vi "LogData.vi"(8 "error in":errorcluster, 10 "Data_Cluster":T1 {"Coil Temperature" format="%.2f"; "Channel 2 (c2)" format="%.3f"; "Channel 1 (c1)" format="%.3f"; "Freqency +45 Deg" format="%.7f"; "Freqency -45 Deg" format="%.7f"; "Freqency 0 Deg" format="%.7f"; "df frequency quotient" format="%.7f"; "Density" format="%.3f"; "Viscosity" format="%.3f"; "Damping Frequency" format="%.2g"; "Resonant Frequency" format="%.2f"; "Temperature" format="%.2f"}) -> (0 "error out":errorcluster)   [LabVIEW 2019, in "SME_Data_Acquisition.lvlib"]
doc: "This even is generated by helper loop to log data.\n_____\nCreated using DQMH Event Scripter 7.0.1.1316."
uses:
  SME_Data_Acquisition.lvlib
  LogData Argument--cluster.ctl
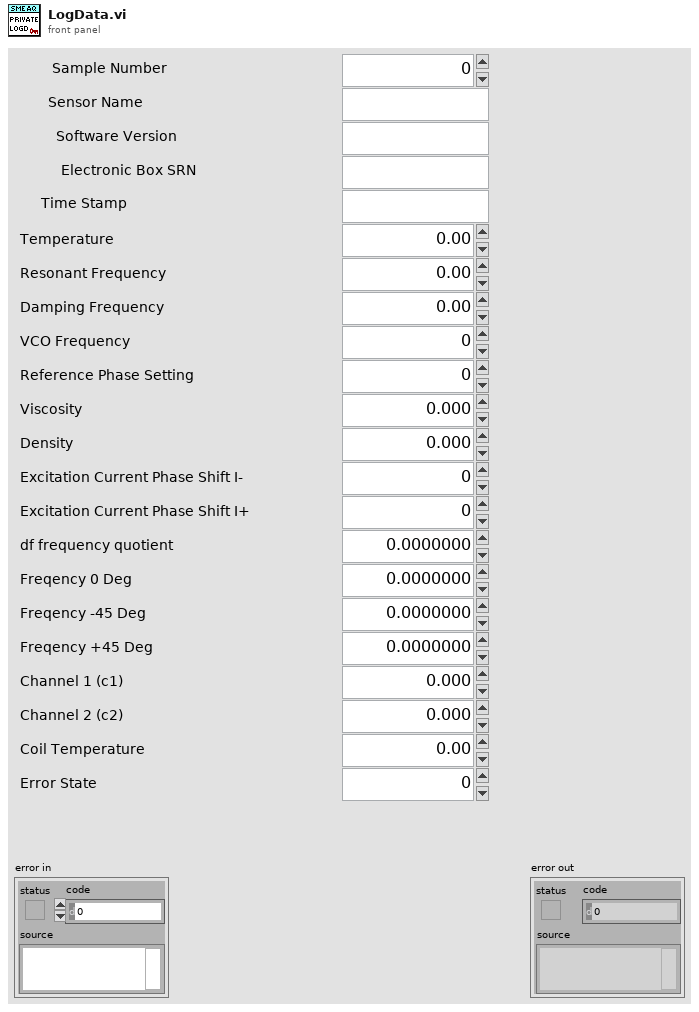
[diagram p1: front panel]
types:
  T1 = cluster{"Sample Number":u16, "Sensor Name":string, "Software Version":string, "Electronic Box SRN":string, "Time Stamp":string, "Temperature":dbl, "Resonant Frequency":dbl, "Damping Frequency":dbl, "VCO Frequency":u16, "Reference Phase Setting":u16, "Viscosity":dbl, "Density":dbl, "Excitation Current Phase Shift I-":u16, "Excitation Current Phase Shift I+":u16, "df frequency quotient":dbl, "Freqency 0 Deg":dbl, "Freqency -45 Deg":dbl, "Freqency +45 Deg":dbl, "Channel 1 (c1)":dbl, "Channel 2 (c2)":dbl, "Coil Temperature":dbl, "Error State":u8}
  T2 = typedef "SME_Data_Acquisition.lvlib/LogData Argument--cluster.ctl" = cluster{"Data_Cluster":cluster{"Sample Number":u16, "Sensor Name":string, "Software Version":string, "Electronic Box SRN":string, "Time Stamp":string, "Temperature":dbl, "Resonant Frequency":dbl, "Damping Frequency":dbl, "VCO Frequency":u16, "Reference Phase Setting":u16, "Viscosity":dbl, "Density":dbl, "Excitation Current Phase Shift I-":u16, "Excitation Current Phase Shift I+":u16, "df frequency quotient":dbl, "Freqency 0 Deg":dbl, "Freqency -45 Deg":dbl, "Freqency +45 Deg":dbl, "Channel 1 (c1)":dbl, "Channel 2 (c2)":dbl, "Coil Temperature":dbl, "Error State":u8}}
  T3 = typedef "SME_Data_Acquisition.lvlib/Request Events--cluster.ctl" = cluster{"Stop Module":refnum<user-event>, "Show Panel":refnum<user-event>, "Hide Panel":refnum<user-event>, "Get Module Execution Status":refnum<user-event>, "Show Diagram":refnum<user-event>, "Private":cluster{"LogData":refnum<user-event>}}
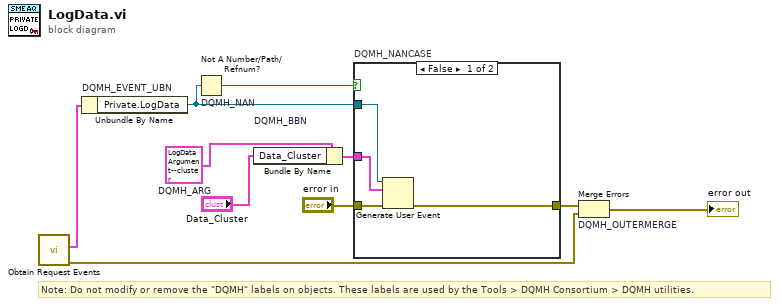
[diagram p0: block diagram]
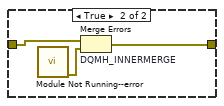
[diagram p2: hidden frame]
diagram:
  w4 = T2 {"Data_Cluster"={"Sample Number"=0, "Sensor Name"="", "Software Version"="", "Electronic Box SRN"="", "Time Stamp"="", "Temperature"=0.0, "Resonant Frequency"=0.0, "Damping Frequency"=0.0, "VCO Frequency"=0, "Reference Phase Setting"=0, "Viscosity"=0.0, "Density"=0.0, "Excitation Current Phase Shift I-"=0, "Excitation Current Phase Shift I+"=0, "df frequency quotient"=0.0, "Freqency 0 Deg"=0.0, "Freqency -45 Deg"=0.0, "Freqency +45 Deg"=0.0, "Channel 1 (c1)"=0.0, "Channel 2 (c2)"=0.0, "Coil Temperature"=0.0, "Error State"=0}}  # DQMH_ARG
  # "Note: Do not modify or remove the \"DQMH\" labels on objects. These labels are used by the Tools > DQMH Consortium > DQMH utilities."
  n1 = call "Obtain Request Events.vi"() -> ("error out"=w2:errorcluster, "SME_Data_Acquisition Request Events"=w1:T3)  [unwired: 10 in]
  n2 = Unbundle By Name "DQMH_EVENT_UBN"(w1) -> ("Private.LogData"=w6:refnum<user-event>)
  n3 = Not A Number/Path/Refnum? "DQMH_NAN"(number/path/refnum=w6) -> (NaN/Path/Refnum?=w7:bool)
  n4 = Bundle By Name "DQMH_BBN"(cluster=w4, "Data_Cluster"="Data_Cluster") -> (w8:T2)
  n5 = case "DQMH_NANCASE" shown="False" w7 {
    tunnel: "error in" -> [w14 w17]
    tunnel: [w13 w16] -> w5
    tunnel: w6 -> [w12 _]
    tunnel: w8 -> [w11 _]
    frame False {
      n6 = Generate User Event(user event=w12, event data cluster=w11, error in=w14) -> (error out=w13:errorcluster)  [unwired: 1 in, 1 out]
    }
    frame True {
      n7 = call "Module Not Running--error.vi"() -> ("error out"=w15:errorcluster)  [unwired: 11 in]
      n8 = Merge Errors "DQMH_INNERMERGE"(w17, w15) -> (w16:errorcluster)
    }
  }
  n9 = Merge Errors "DQMH_OUTERMERGE"(w5, w2) -> (→"error out":errorcluster)
